vi "Timer.vi"(7 "Timer States":T1, 11 "Time to timeout":u32) -> (3 "Timeout":bool)   [LabVIEW 2017]
uses:
  Type Definitions/Timer States.ctl
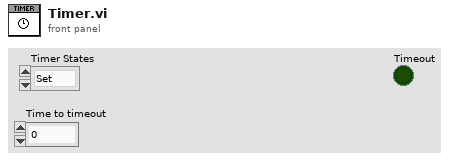
[diagram p1: front panel]
types:
  T1 = typedef "Timer States.ctl" = enum16{"Set", "Get"}
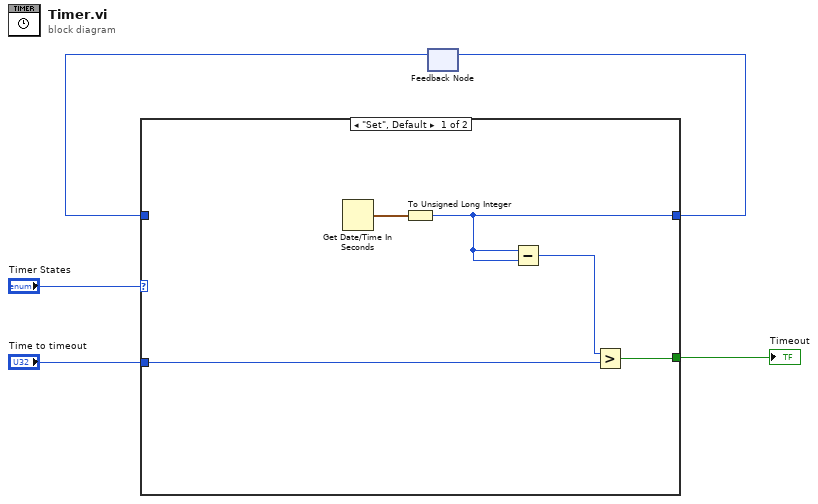
[diagram p0: block diagram]
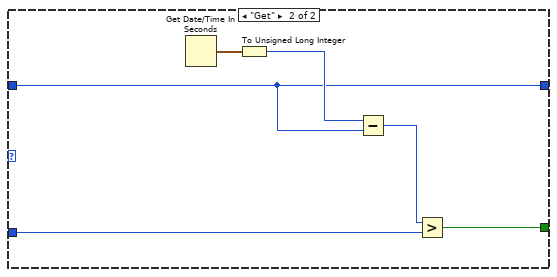
[diagram p2: hidden frame]
diagram:
  n1 = feedback #1() -> (w2:u32)  [unwired: 1 in]
  n2 = case shown="\"Set\", Default" "Timer States" {
    tunnel: "Time to timeout" -> [w6 w13]
    tunnel: [w9 w14] -> w3
    tunnel: w2 -> [_ w14]
    tunnel: [w7 w11] -> w1
    frame "Set", Default {
      n3 = Get Date/Time In Seconds() -> (seconds since 1Jan1904=w10:timestamp)
      n4 = To Unsigned Long Integer(number=w10) -> (unsigned 32bit integer=w9:u32)
      n5 = Subtract(x=w9, y=w9) -> (x-y=w8:u32)
      n6 = Greater?(x=w8, y=w6) -> (0:w7:bool)
    }
    frame "Get" {
      n7 = Get Date/Time In Seconds() -> (seconds since 1Jan1904=w16:timestamp)
      n8 = To Unsigned Long Integer(number=w16) -> (unsigned 32bit integer=w15:u32)
      n9 = Subtract(x=w15, y=w14) -> (x-y=w12:u32)
      n10 = Greater?(x=w12, y=w13) -> (0:w11:bool)
    }
  }
  "Timeout" <- w1
  n11 = feedback-in #1(w3) -> ()
